vi "Notifiers.vi"() -> ()   [LabVIEW 2019]
panel:
  in  "Slide":dbl(slide) scale=0.0..10.0
  out "Slider Value":dbl
  in  "Generate 2":bool
  in  "Loop 3 Stop":bool
  in  "Loop 2 Stop":bool
  in  "Generate":bool
  in  "Loop 1 Stop":bool
  out "Number Displayed in Loop 3":dbl
  out "Number Displayed in Loop 2":dbl
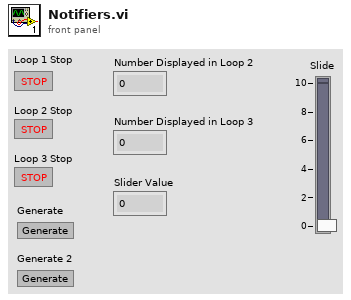
[diagram p1: front panel]
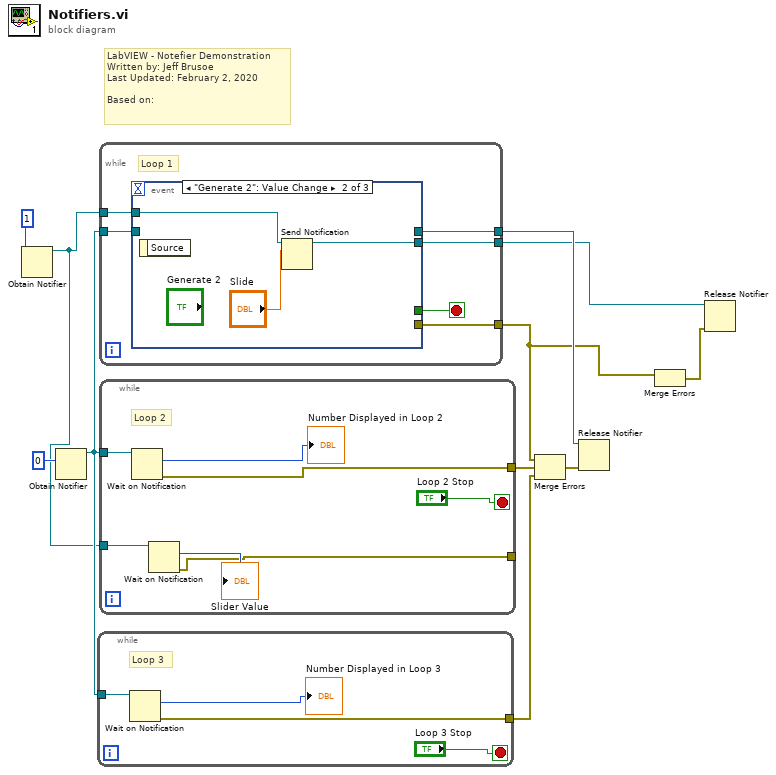
[diagram p0: block diagram]
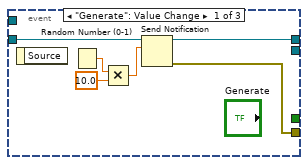
[diagram p2: hidden frame]
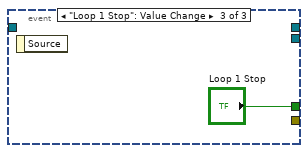
[diagram p3: hidden frame]
diagram:
  # "LabVIEW - Notefier Demonstration\nWritten by: Jeff Brusoe\nLast Updated: February 2, 2020\n\nBased on:"
  n1 = Obtain Notifier(notification data type=1) -> (notifier out=w3:refnum<notifier>)  [unwired: 3 in, 2 out]
  n2 = Obtain Notifier(notification data type=0) -> (notifier out=w9:refnum<notifier>)  [unwired: 3 in, 2 out]
  n3 = while {
    tunnel: w9 -> [w15]
    tunnel: [w12] -> w7
    stop <- "Loop 3 Stop" stop-if-true
    # "Loop 3"
    n4 = Wait on Notification(notifier=w15) -> (notification=→"Number Displayed in Loop 3":i32, error out=w12:errorcluster)  [unwired: 3 in, 2 out]
  }
  n5 = while {
    tunnel: w9 -> [w21]
    tunnel: [w20] -> w10
    tunnel: [w18] -> w2
    tunnel: w3 -> [w17]
    tunnel: [w16] -> w4
    stop <- w19 stop-if-true
    # "Loop 1"
    n6 = event shown="[1] \"Generate 2\": Value Change" {
      selector: _ -> [_ _ _]
      dyn-events: _ -> [_ _ _]
      timeout: _ -> [_ _ _]
      tunnel: w21 -> [w24 _ _]
      tunnel: [w23 _ _] -> w20
      tunnel: [_ _ "Loop 1 Stop"] -> w19
      tunnel: [w22 _ _] -> w18
      tunnel: w17 -> [_ w29 _]
      tunnel: [_ w30 _] -> w16
      event "Generate": Value Change {
        n7 = event-data() -> ()  [unwired: 1 in, 1 out]
        n8 = Random Number (0-1)() -> (number: 0 to 1=w27:dbl)
        n9 = Multiply(x=w27, y=10.0) -> (x*y=w25:dbl)
        n10 = Send Notification(notification=w25, notifier=w24) -> (notifier out=w23:refnum<notifier>, error out=w22:errorcluster)  [unwired: 1 in]
      }
      event "Generate 2": Value Change {
        n11 = event-data() -> ()  [unwired: 1 in, 1 out]
        n12 = Send Notification(notification="Slide", notifier=w29) -> (notifier out=w30:refnum<notifier>)  [unwired: 1 in, 1 out]
      }
      event "Loop 1 Stop": Value Change {
        n13 = event-data() -> ()  [unwired: 1 in, 1 out]
      }
    }
  }
  n14 = while {
    tunnel: w9 -> [w38]
    tunnel: [w35] -> w8
    tunnel: w3 -> [w34]
    tunnel: [w32] -> _
    stop <- "Loop 2 Stop" stop-if-true
    # "Loop 2"
    n15 = Wait on Notification(notifier=w38) -> (notification=→"Number Displayed in Loop 2":i32, error out=w35:errorcluster)  [unwired: 3 in, 2 out]
    n16 = Wait on Notification(notifier=w34) -> (notification=→"Slider Value":i32, error out=w32:errorcluster)  [unwired: 3 in, 2 out]
  }
  n17 = Merge Errors(w2, w8, w7) -> (w6:errorcluster)
  n18 = Release Notifier(notifier=w10, error in (no error)=w6) -> ()  [unwired: 1 in, 3 out]
  n19 = Merge Errors(w2) -> (w1:errorcluster)  [unwired: 1 in]
  n20 = Release Notifier(notifier=w4, error in (no error)=w1) -> ()  [unwired: 1 in, 3 out]
